vi "Update PID.vi"(8 "error in (no error)":errorcluster, 10 "ctl":cluster{"p":dbl, "i":dbl, "d":dbl}, 11 "TEC in":refnum<class "TEC.lvclass">) -> (0 "error out":errorcluster, 3 "TEC out":refnum<class "TEC.lvclass">)   [LabVIEW 2015, in "Generic TEC.lvlib" / "TEC.lvclass"]
uses:
  TEC.lvclass
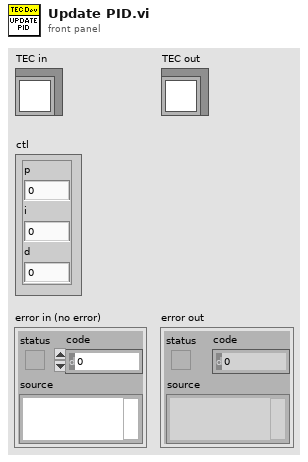
[diagram p1: front panel]
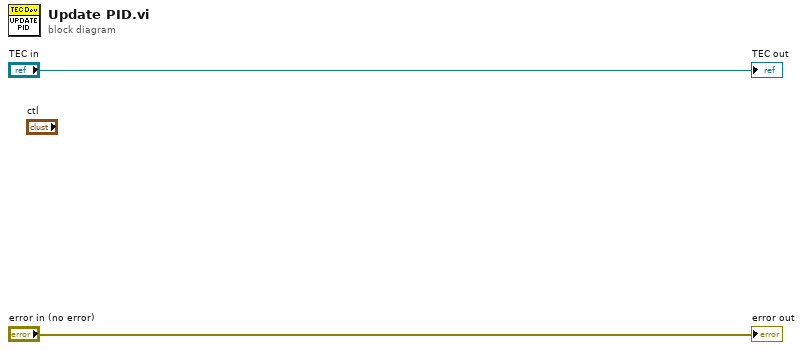
[diagram p0: block diagram]
diagram:
  "error out" <- "error in (no error)"
  "TEC out" <- "TEC in"
